vi "FGGA TCP Packet_v3.2.vi"(0 "ID":string, 5 "Version":string, 7 "TCP Packet In":string, 9 "utc_time":u32, 12 "Data Array":string[](array[string])) -> (8 "TCP Binary Packet":string)   [LabVIEW 2014]
panel:
  out "array":string[](array[string])
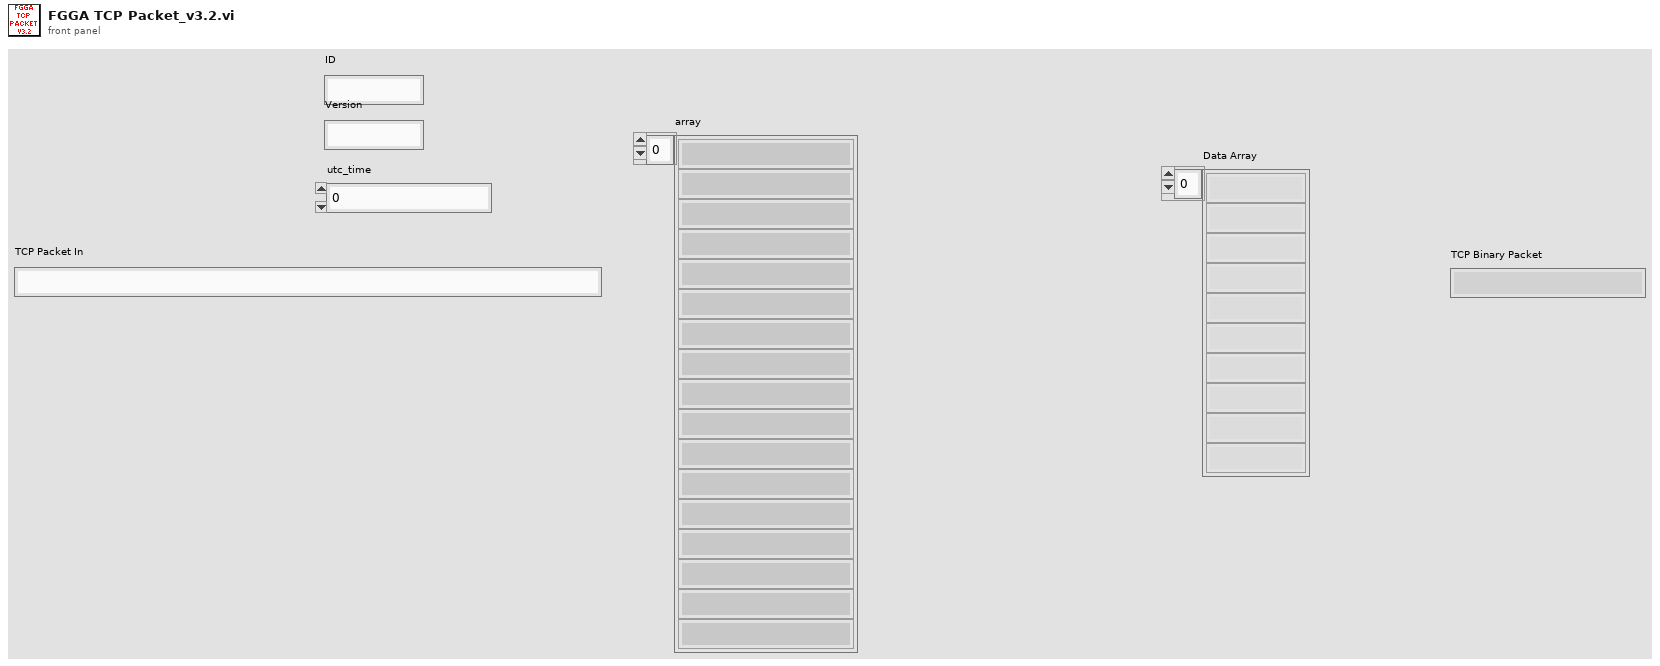
[diagram p1: front panel]
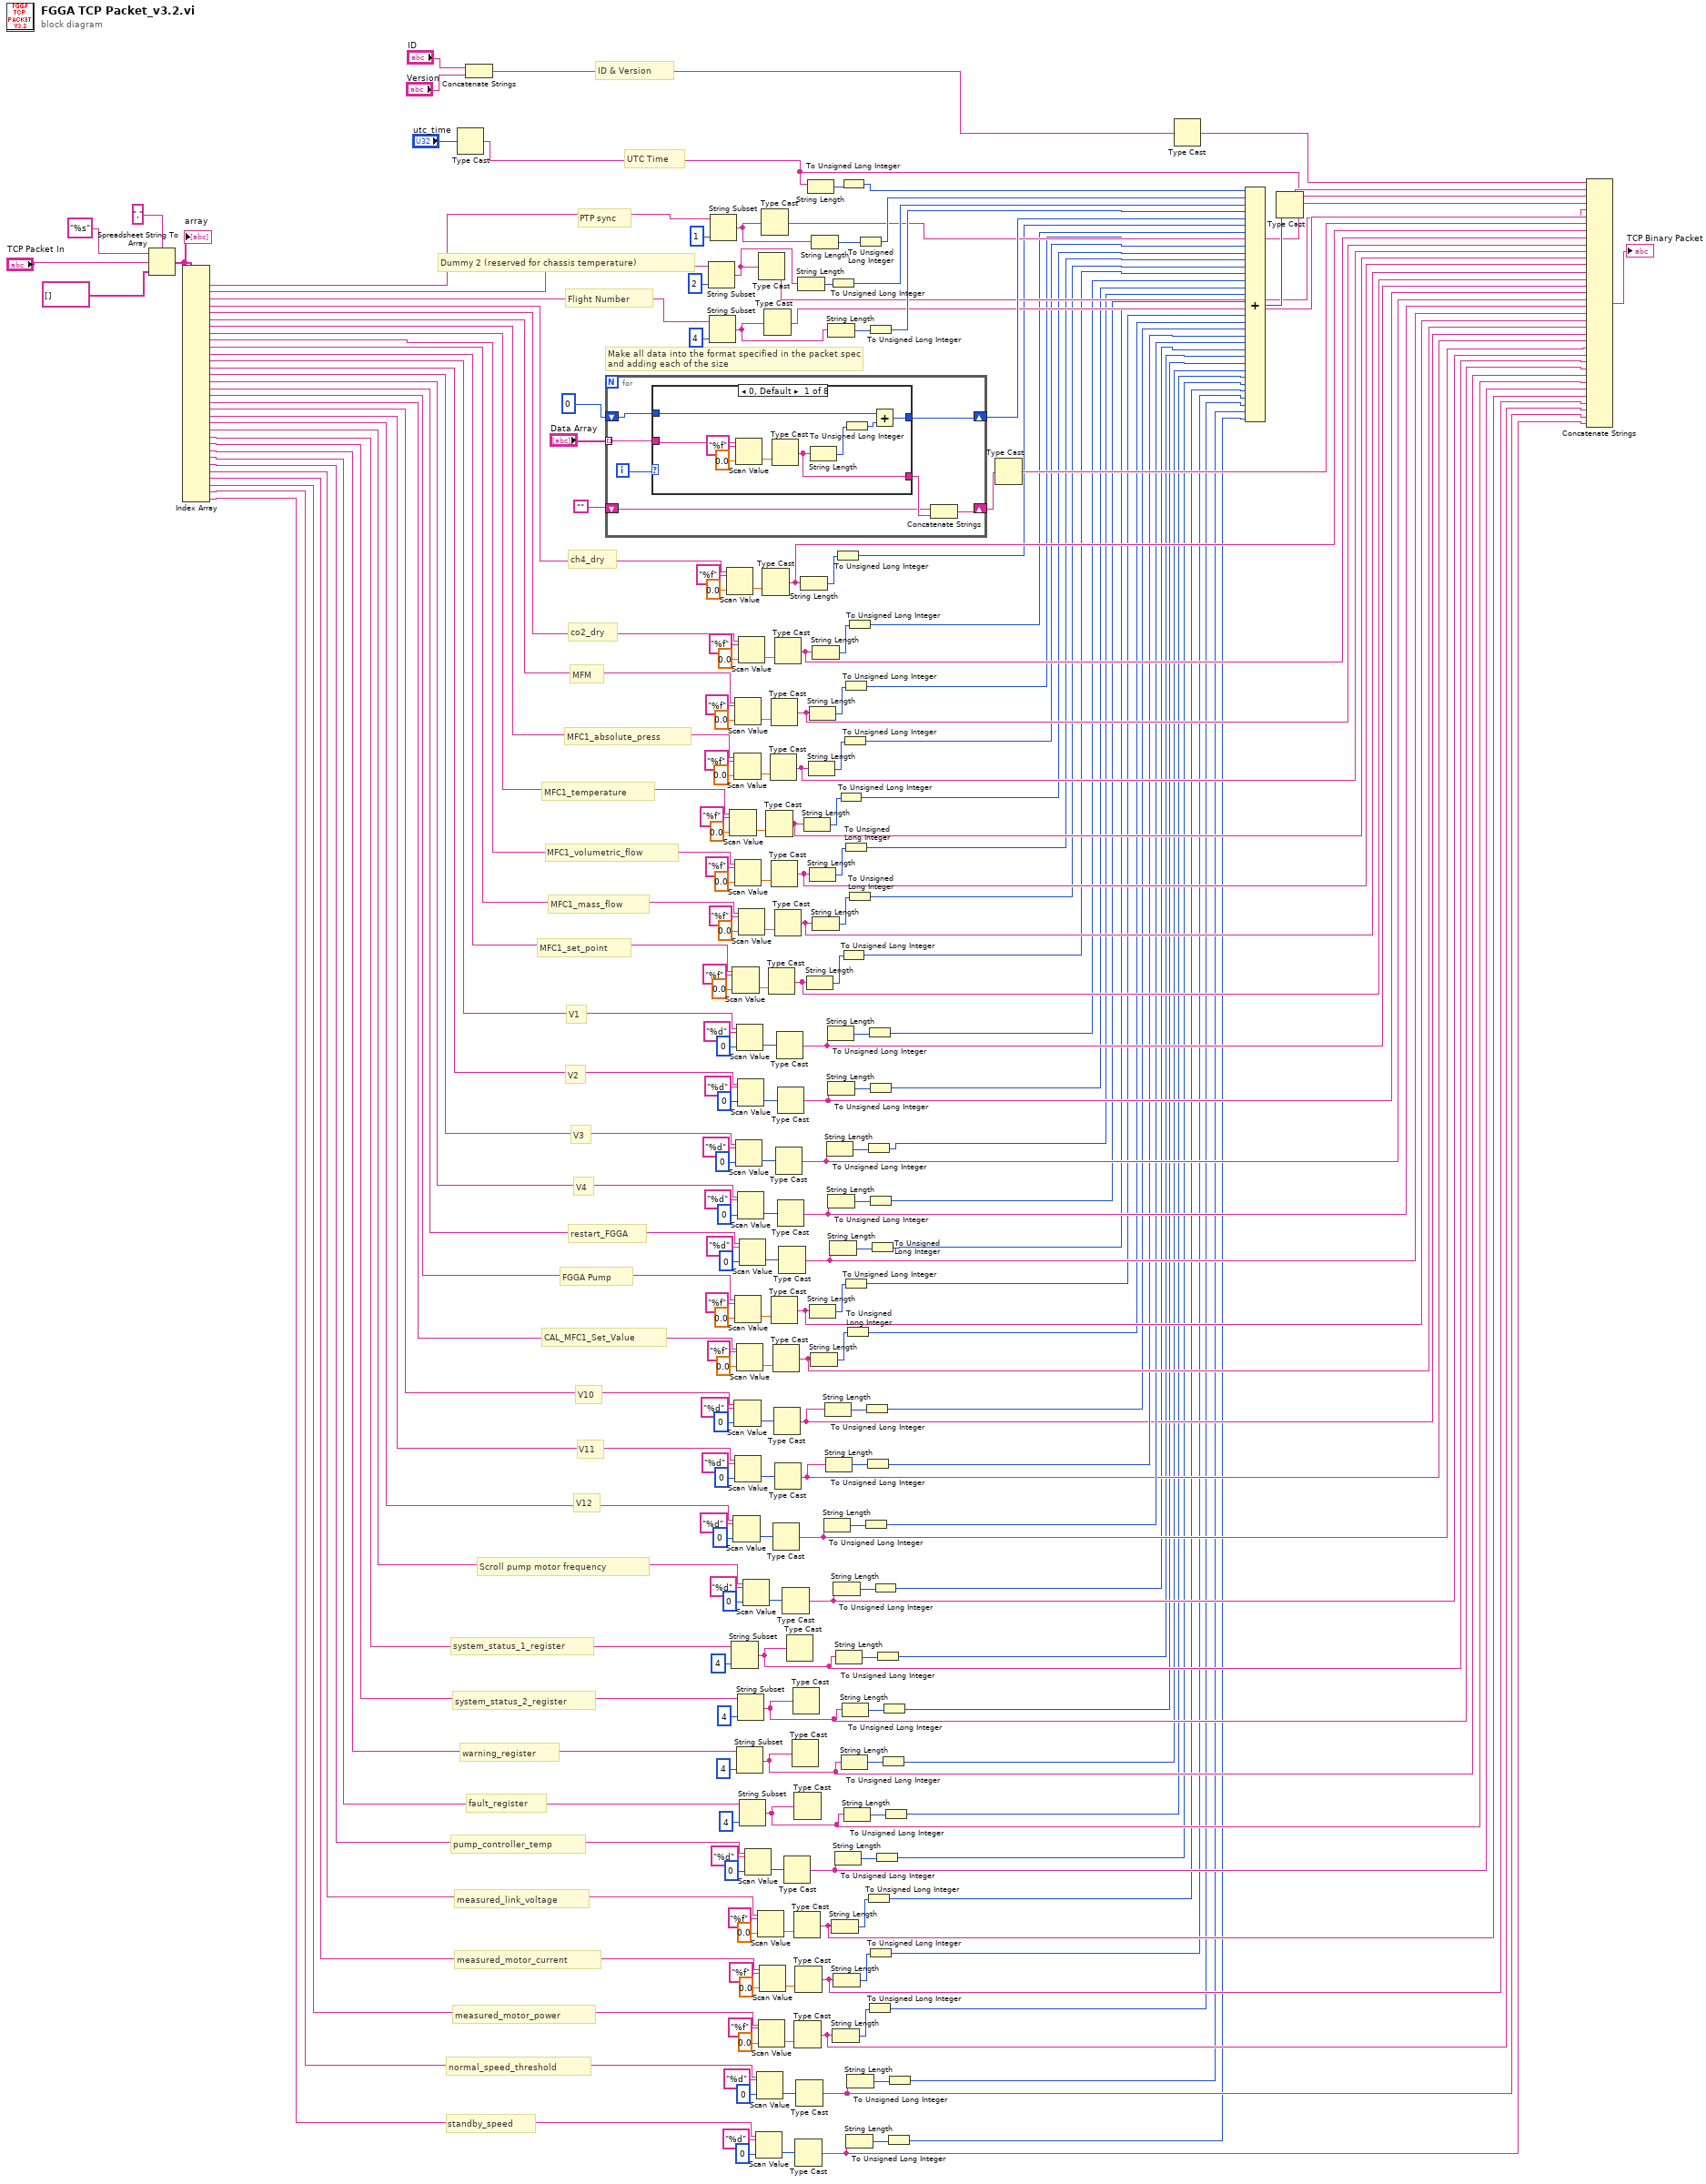
[diagram p0: block diagram]
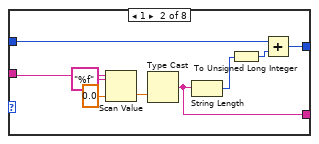
[diagram p2: hidden frame]
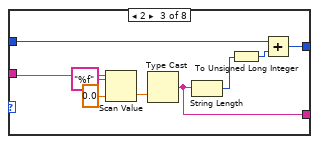
[diagram p3: hidden frame]
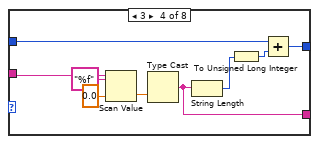
[diagram p4: hidden frame]
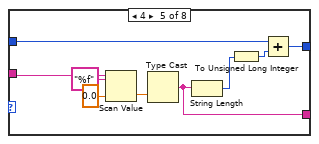
[diagram p5: hidden frame]
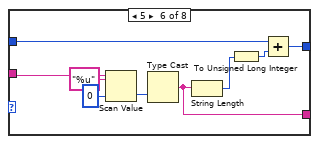
[diagram p6: hidden frame]
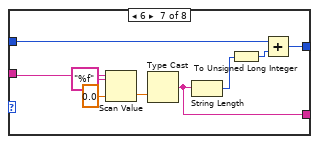
[diagram p7: hidden frame]
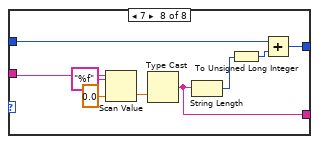
[diagram p8: hidden frame]
diagram:
  # "standby_speed"
  # "normal_speed_threshold"
  # "measured_motor_power"
  # "measured_motor_current"
  # "measured_link_voltage"
  # "pump_controller_temp"
  # "fault_register"
  # "warning_register"
  # "system_status_2_register"
  # "system_status_1_register"
  # "Scroll pump motor frequency"
  # "V12"
  # "V11"
  # "V10"
  # "PTP sync"
  # "CAL_MFC1_Set_Value"
  # "FGGA Pump"
  # "restart_FGGA"
  # "V4"
  # "V3"
  # "V2"
  # "V1"
  # "MFC1_set_point"
  # "MFC1_mass_flow"
  # "MFC1_volumetric_flow"
  # "MFC1_temperature"
  # "MFC1_absolute_press"
  # "MFM"
  # "co2_dry"
  # "ch4_dry"
  # "Flight Number"
  # "Dummy 2 (reserved for chassis temperature)"
  # "UTC Time"
  # "ID & Version"
  # "Make all data into the format specified in the packet spec\nand adding each of the size"
  n1 = Spreadsheet String To Array(delimiter (Tab)=",", format string="%s", spreadsheet string="TCP Packet In", array type (2D Dbl)=string[] []) -> (array=w192:string[])
  "array" <- w192
  n2 = Index Array(array=w192) -> (element #1=w191:string, element #2=w190:string, element #3=w189:string, element #4=w188:string, element #5=w187:string, element #6=w162:string, element #7=w159:string, element #8=w156:string, element #9=w153:string, element #10=w150:string, element #11=w147:string, element #12=w140:string, element #13=w133:string, element #14=w110:string, element #15=w107:string, element #16=w104:string, element #17=w101:string, element #18=w98:string, element #19=w78:string, element #20=w77:string, element #21=w76:string, element #22=w33:string, element #23=w32:string, element #24=w31:string, element #25=w30:string, element #26=w29:string, element #27=w28:string, element #28=w27:string, element #29=w26:string, element #30=w25:string, element #31=w24:string, element #32=w23:string)  [unwired: 32 in]
  n3 = Type Cast(x="utc_time") -> (*(type *) &x=w91:string)  [unwired: 1 in]
  n4 = Concatenate Strings("ID", "Version") -> (w93:string)
  n5 = for {
    tunnel: "Data Array" -> [w241] mode=indexing
    shift-right: [w239] -> w223
    shift-left: u32 0 -> [w240]
    shift-right: [w238] -> w212
    shift-left: "" -> [w236]
    i -> [w242]
    n6 = case shown="0, Default" w242 {
      tunnel: w241 -> [w249 w258 w267 w276 w285 w294 w303 w312]
      tunnel: w240 -> [w247 w256 w265 w274 w283 w292 w301 w310]
      tunnel: [w244 w253 w262 w271 w280 w289 w298 w307] -> w239
      tunnel: [w243 w252 w261 w270 w279 w288 w297 w306] -> w237
      frame 0, Default {
        n7 = Scan Value(string=w249, format string="%f", default (0 dbl)=sgl 0.0 ("default (0 I32)")) -> (value=w251:sgl)  [unwired: 1 out]
        n8 = Type Cast(x=w251) -> (*(type *) &x=w243:string)  [unwired: 1 in]
        n9 = String Length(string=w243) -> (length=w246:i32)
        n10 = To Unsigned Long Integer(number=w246) -> (unsigned 32bit integer=w245:u32)
        n11 = Add(x=w247, y=w245) -> (x+y=w244:u32)
      }
      frame 1 {
        n12 = Scan Value(string=w258, format string="%f", default (0 dbl)=sgl 0.0 ("default (0 I32)")) -> (value=w260:sgl)  [unwired: 1 out]
        n13 = Type Cast(x=w260) -> (*(type *) &x=w252:string)  [unwired: 1 in]
        n14 = String Length(string=w252) -> (length=w255:i32)
        n15 = To Unsigned Long Integer(number=w255) -> (unsigned 32bit integer=w254:u32)
        n16 = Add(x=w256, y=w254) -> (x+y=w253:u32)
      }
      frame 2 {
        n17 = Scan Value(string=w267, format string="%f", default (0 dbl)=sgl 0.0 ("default (0 I32)")) -> (value=w269:sgl)  [unwired: 1 out]
        n18 = Type Cast(x=w269) -> (*(type *) &x=w261:string)  [unwired: 1 in]
        n19 = String Length(string=w261) -> (length=w264:i32)
        n20 = To Unsigned Long Integer(number=w264) -> (unsigned 32bit integer=w263:u32)
        n21 = Add(x=w265, y=w263) -> (x+y=w262:u32)
      }
      frame 3 {
        n22 = Scan Value(string=w276, format string="%f", default (0 dbl)=sgl 0.0 ("default (0 I32)")) -> (value=w278:sgl)  [unwired: 1 out]
        n23 = Type Cast(x=w278) -> (*(type *) &x=w270:string)  [unwired: 1 in]
        n24 = String Length(string=w270) -> (length=w273:i32)
        n25 = To Unsigned Long Integer(number=w273) -> (unsigned 32bit integer=w272:u32)
        n26 = Add(x=w274, y=w272) -> (x+y=w271:u32)
      }
      frame 4 {
        n27 = Scan Value(string=w285, format string="%f", default (0 dbl)=sgl 0.0 ("default (0 I32)")) -> (value=w287:sgl)  [unwired: 1 out]
        n28 = Type Cast(x=w287) -> (*(type *) &x=w279:string)  [unwired: 1 in]
        n29 = String Length(string=w279) -> (length=w282:i32)
        n30 = To Unsigned Long Integer(number=w282) -> (unsigned 32bit integer=w281:u32)
        n31 = Add(x=w283, y=w281) -> (x+y=w280:u32)
      }
      frame 5 {
        n32 = Scan Value(string=w294, format string="%u", default (0 dbl)=u16 0 ("default (0 I32)")) -> (value=w296:u16)  [unwired: 1 out]
        n33 = Type Cast(x=w296) -> (*(type *) &x=w288:string)  [unwired: 1 in]
        n34 = String Length(string=w288) -> (length=w291:i32)
        n35 = To Unsigned Long Integer(number=w291) -> (unsigned 32bit integer=w290:u32)
        n36 = Add(x=w292, y=w290) -> (x+y=w289:u32)
      }
      frame 6 {
        n37 = Scan Value(string=w303, format string="%f", default (0 dbl)=sgl 0.0 ("default (0 I32)")) -> (value=w305:sgl)  [unwired: 1 out]
        n38 = Type Cast(x=w305) -> (*(type *) &x=w297:string)  [unwired: 1 in]
        n39 = String Length(string=w297) -> (length=w300:i32)
        n40 = To Unsigned Long Integer(number=w300) -> (unsigned 32bit integer=w299:u32)
        n41 = Add(x=w301, y=w299) -> (x+y=w298:u32)
      }
      frame 7 {
        n42 = Scan Value(string=w312, format string="%f", default (0 dbl)=sgl 0.0 ("default (0 I32)")) -> (value=w314:sgl)  [unwired: 1 out]
        n43 = Type Cast(x=w314) -> (*(type *) &x=w306:string)  [unwired: 1 in]
        n44 = String Length(string=w306) -> (length=w309:i32)
        n45 = To Unsigned Long Integer(number=w309) -> (unsigned 32bit integer=w308:u32)
        n46 = Add(x=w310, y=w308) -> (x+y=w307:u32)
      }
    }
    n47 = Concatenate Strings(w236, w237) -> (w238:string)
  }
  n48 = String Subset(string=w190, length (rest)=2 ("length (rest)")) -> (substring=w210:string)  [unwired: 1 in]
  n49 = String Subset(string=w189, length (rest)=4 ("length (rest)")) -> (substring=w216:string)  [unwired: 1 in]
  n50 = String Subset(string=w191, length (rest)=1 ("length (rest)")) -> (substring=w219:string)  [unwired: 1 in]
  n51 = Scan Value(string=w188, format string="%f", default (0 dbl)=sgl 0.0 ("default (0 I32)")) -> (value=w208:sgl)  [unwired: 1 out]
  n52 = Scan Value(string=w156, format string="%f", default (0 dbl)=sgl 0.0 ("default (0 I32)")) -> (value=w178:sgl)  [unwired: 1 out]
  n53 = String Subset(string=w32, length (rest)=4 ("length (rest)")) -> (substring=w19:string)  [unwired: 1 in]
  n54 = Scan Value(string=w147, format string="%f", default (0 dbl)=sgl 0.0 ("default (0 I32)")) -> (value=w166:sgl)  [unwired: 1 out]
  n55 = Scan Value(string=w76, format string="%d", default (0 dbl)=u16 0 ("default (0 I32)")) -> (value=w79:u16)  [unwired: 1 out]
  n56 = Scan Value(string=w159, format string="%f", default (0 dbl)=sgl 0.0 ("default (0 I32)")) -> (value=w182:sgl)  [unwired: 1 out]
  n57 = Scan Value(string=w78, format string="%d", default (0 dbl)=u16 0 ("default (0 I32)")) -> (value=w87:u16)  [unwired: 1 out]
  n58 = Scan Value(string=w162, format string="%f", default (0 dbl)=sgl 0.0 ("default (0 I32)")) -> (value=w186:sgl)  [unwired: 1 out]
  n59 = Scan Value(string=w153, format string="%f", default (0 dbl)=sgl 0.0 ("default (0 I32)")) -> (value=w174:sgl)  [unwired: 1 out]
  n60 = Scan Value(string=w101, format string="%f", default (0 dbl)=sgl 0.0 ("default (0 I32)")) -> (value=w118:sgl)  [unwired: 1 out]
  n61 = Scan Value(string=w77, format string="%d", default (0 dbl)=u16 0 ("default (0 I32)")) -> (value=w83:u16)  [unwired: 1 out]
  n62 = Scan Value(string=w110, format string="%d", default (0 dbl)=u16 0 ("default (0 I32)")) -> (value=w127:u16)  [unwired: 1 out]
  n63 = Scan Value(string=w140, format string="%d", default (0 dbl)=u16 0 ("default (0 I32)")) -> (value=w141:u16)  [unwired: 1 out]
  n64 = Scan Value(string=w98, format string="%f", default (0 dbl)=sgl 0.0 ("default (0 I32)")) -> (value=w114:sgl)  [unwired: 1 out]
  n65 = String Subset(string=w30, length (rest)=4 ("length (rest)")) -> (substring=w15:string)  [unwired: 1 in]
  n66 = Scan Value(string=w133, format string="%d", default (0 dbl)=u16 0 ("default (0 I32)")) -> (value=w134:u16)  [unwired: 1 out]
  n67 = Scan Value(string=w107, format string="%d", default (0 dbl)=u16 0 ("default (0 I32)")) -> (value=w123:u16)  [unwired: 1 out]
  n68 = String Subset(string=w31, length (rest)=4 ("length (rest)")) -> (substring=w17:string)  [unwired: 1 in]
  n69 = Scan Value(string=w187, format string="%f", default (0 dbl)=sgl 0.0 ("default (0 I32)")) -> (value=w202:sgl)  [unwired: 1 out]
  n70 = Scan Value(string=w150, format string="%f", default (0 dbl)=sgl 0.0 ("default (0 I32)")) -> (value=w170:sgl)  [unwired: 1 out]
  n71 = Scan Value(string=w104, format string="%d", default (0 dbl)=u16 0 ("default (0 I32)")) -> (value=w119:u16)  [unwired: 1 out]
  n72 = String Subset(string=w29, length (rest)=4 ("length (rest)")) -> (substring=w13:string)  [unwired: 1 in]
  n73 = Scan Value(string=w33, format string="%d", default (0 dbl)=u16 0 ("default (0 I32)")) -> (value=w66:u16)  [unwired: 1 out]
  n74 = Scan Value(string=w28, format string="%d", default (0 dbl)=u16 0 ("default (0 I32)")) -> (value=w54:u16)  [unwired: 1 out]
  n75 = Scan Value(string=w23, format string="%d", default (0 dbl)=u16 0 ("default (0 I32)")) -> (value=w34:u16)  [unwired: 1 out]
  n76 = Scan Value(string=w24, format string="%d", default (0 dbl)=u16 0 ("default (0 I32)")) -> (value=w38:u16)  [unwired: 1 out]
  n77 = Scan Value(string=w27, format string="%f", default (0 dbl)=sgl 0.0 ("default (0 I32)")) -> (value=w53:sgl)  [unwired: 1 out]
  n78 = Type Cast(x=w210) -> (*(type *) &x=w209:string)  [unwired: 1 in]
  n79 = Scan Value(string=w25, format string="%f", default (0 dbl)=sgl 0.0 ("default (0 I32)")) -> (value=w45:sgl)  [unwired: 1 out]
  n80 = Scan Value(string=w26, format string="%f", default (0 dbl)=sgl 0.0 ("default (0 I32)")) -> (value=w49:sgl)  [unwired: 1 out]
  n81 = Type Cast(x=w219) -> (*(type *) &x=w218:string)  [unwired: 1 in]
  n82 = Type Cast(x=w208) -> (*(type *) &x=w204:string)  [unwired: 1 in]
  n83 = Type Cast(x=w216) -> (*(type *) &x=w217:string)  [unwired: 1 in]
  n84 = Type Cast(x=w178) -> (*(type *) &x=w154:string)  [unwired: 1 in]
  n85 = Type Cast(x=w166) -> (*(type *) &x=w145:string)  [unwired: 1 in]
  n86 = Type Cast(x=w182) -> (*(type *) &x=w157:string)  [unwired: 1 in]
  n87 = Type Cast(x=w186) -> (*(type *) &x=w160:string)  [unwired: 1 in]
  n88 = Type Cast(x=w174) -> (*(type *) &x=w151:string)  [unwired: 1 in]
  n89 = Type Cast(x=w118) -> (*(type *) &x=w99:string)  [unwired: 1 in]
  n90 = Type Cast(x=w114) -> (*(type *) &x=w96:string)  [unwired: 1 in]
  n91 = Type Cast(x=w79) -> (*(type *) &x=w70:string)  [unwired: 1 in]
  n92 = Type Cast(x=w87) -> (*(type *) &x=w72:string)  [unwired: 1 in]
  n93 = Type Cast(x=w202) -> (*(type *) &x=w197:string)  [unwired: 1 in]
  n94 = Type Cast(x=w170) -> (*(type *) &x=w148:string)  [unwired: 1 in]
  n95 = Type Cast(x=w83) -> (*(type *) &x=w71:string)  [unwired: 1 in]
  n96 = Type Cast(x=w127) -> (*(type *) &x=w108:string)  [unwired: 1 in]
  n97 = Type Cast(x=w141) -> (*(type *) &x=w138:string)  [unwired: 1 in]
  n98 = Type Cast(x=w134) -> (*(type *) &x=w131:string)  [unwired: 1 in]
  n99 = Type Cast(x=w123) -> (*(type *) &x=w105:string)  [unwired: 1 in]
  n100 = Type Cast(x=w119) -> (*(type *) &x=w102:string)  [unwired: 1 in]
  n101 = Type Cast(x=w66) -> (*(type *) &x=w21:string)  [unwired: 1 in]
  n102 = Type Cast(x=w54) -> (*(type *) &x=w11:string)  [unwired: 1 in]
  n103 = Type Cast(x=w19) -> ()  [unwired: 1 in, 1 out]
  n104 = Type Cast(x=w15) -> ()  [unwired: 1 in, 1 out]
  n105 = Type Cast(x=w17) -> ()  [unwired: 1 in, 1 out]
  n106 = Type Cast(x=w53) -> (*(type *) &x=w9:string)  [unwired: 1 in]
  n107 = Type Cast(x=w13) -> ()  [unwired: 1 in, 1 out]
  n108 = Type Cast(x=w45) -> (*(type *) &x=w5:string)  [unwired: 1 in]
  n109 = Type Cast(x=w49) -> (*(type *) &x=w7:string)  [unwired: 1 in]
  n110 = Type Cast(x=w34) -> (*(type *) &x=w1:string)  [unwired: 1 in]
  n111 = Type Cast(x=w38) -> (*(type *) &x=w3:string)  [unwired: 1 in]
  n112 = String Length(string=w210) -> (length=w230:i32)
  n113 = String Length(string=w204) -> (length=w205:i32)
  n114 = String Length(string=w154) -> (length=w175:i32)
  n115 = String Length(string=w145) -> (length=w163:i32)
  n116 = String Length(string=w91) -> (length=w235:i32)
  n117 = String Length(string=w157) -> (length=w179:i32)
  n118 = String Length(string=w160) -> (length=w183:i32)
  n119 = String Length(string=w151) -> (length=w171:i32)
  n120 = String Length(string=w99) -> (length=w115:i32)
  n121 = String Length(string=w96) -> (length=w111:i32)
  n122 = String Length(string=w219) -> (length=w232:i32)
  n123 = String Length(string=w197) -> (length=w199:i32)
  n124 = String Length(string=w148) -> (length=w167:i32)
  n125 = String Length(string=w70) -> (length=w82:i32)
  n126 = String Length(string=w72) -> (length=w90:i32)
  n127 = String Length(string=w71) -> (length=w86:i32)
  n128 = String Length(string=w108) -> (length=w130:i32)
  n129 = String Length(string=w138) -> (length=w144:i32)
  n130 = String Length(string=w216) -> (length=w227:i32)
  n131 = String Length(string=w131) -> (length=w137:i32)
  n132 = String Length(string=w105) -> (length=w126:i32)
  n133 = To Unsigned Long Integer(number=w230) -> (unsigned 32bit integer=w229:u32)
  n134 = String Length(string=w102) -> (length=w122:i32)
  n135 = String Length(string=w9) -> (length=w50:i32)
  n136 = String Length(string=w5) -> (length=w42:i32)
  n137 = String Length(string=w21) -> (length=w69:i32)
  n138 = String Length(string=w7) -> (length=w46:i32)
  n139 = To Unsigned Long Integer(number=w205) -> (unsigned 32bit integer=w203:u32)
  n140 = String Length(string=w11) -> (length=w57:i32)
  n141 = String Length(string=w19) -> (length=w64:i32)
  n142 = To Unsigned Long Integer(number=w175) -> (unsigned 32bit integer=w155:u32)
  n143 = To Unsigned Long Integer(number=w235) -> (unsigned 32bit integer=w234:u32)
  n144 = To Unsigned Long Integer(number=w163) -> (unsigned 32bit integer=w146:u32)
  n145 = String Length(string=w15) -> (length=w60:i32)
  n146 = To Unsigned Long Integer(number=w179) -> (unsigned 32bit integer=w158:u32)
  n147 = String Length(string=w17) -> (length=w62:i32)
  n148 = To Unsigned Long Integer(number=w183) -> (unsigned 32bit integer=w161:u32)
  n149 = To Unsigned Long Integer(number=w171) -> (unsigned 32bit integer=w152:u32)
  n150 = To Unsigned Long Integer(number=w115) -> (unsigned 32bit integer=w100:u32)
  n151 = String Length(string=w13) -> (length=w58:i32)
  n152 = To Unsigned Long Integer(number=w111) -> (unsigned 32bit integer=w97:u32)
  n153 = To Unsigned Long Integer(number=w199) -> (unsigned 32bit integer=w198:u32)
  n154 = To Unsigned Long Integer(number=w167) -> (unsigned 32bit integer=w149:u32)
  n155 = String Length(string=w1) -> (length=w37:i32)
  n156 = String Length(string=w3) -> (length=w41:i32)
  n157 = To Unsigned Long Integer(number=w232) -> (unsigned 32bit integer=w231:u32)
  n158 = To Unsigned Long Integer(number=w82) -> (unsigned 32bit integer=w73:u32)
  n159 = To Unsigned Long Integer(number=w90) -> (unsigned 32bit integer=w75:u32)
  n160 = To Unsigned Long Integer(number=w86) -> (unsigned 32bit integer=w74:u32)
  n161 = To Unsigned Long Integer(number=w130) -> (unsigned 32bit integer=w109:u32)
  n162 = To Unsigned Long Integer(number=w50) -> (unsigned 32bit integer=w10:u32)
  n163 = To Unsigned Long Integer(number=w144) -> (unsigned 32bit integer=w139:u32)
  n164 = To Unsigned Long Integer(number=w42) -> (unsigned 32bit integer=w6:u32)
  n165 = To Unsigned Long Integer(number=w227) -> (unsigned 32bit integer=w226:u32)
  n166 = To Unsigned Long Integer(number=w137) -> (unsigned 32bit integer=w132:u32)
  n167 = To Unsigned Long Integer(number=w126) -> (unsigned 32bit integer=w106:u32)
  n168 = To Unsigned Long Integer(number=w46) -> (unsigned 32bit integer=w8:u32)
  n169 = To Unsigned Long Integer(number=w122) -> (unsigned 32bit integer=w103:u32)
  n170 = To Unsigned Long Integer(number=w69) -> (unsigned 32bit integer=w22:u32)
  n171 = To Unsigned Long Integer(number=w57) -> (unsigned 32bit integer=w12:u32)
  n172 = To Unsigned Long Integer(number=w64) -> (unsigned 32bit integer=w20:u32)
  n173 = To Unsigned Long Integer(number=w60) -> (unsigned 32bit integer=w16:u32)
  n174 = To Unsigned Long Integer(number=w62) -> (unsigned 32bit integer=w18:u32)
  n175 = To Unsigned Long Integer(number=w58) -> (unsigned 32bit integer=w14:u32)
  n176 = To Unsigned Long Integer(number=w37) -> (unsigned 32bit integer=w2:u32)
  n177 = To Unsigned Long Integer(number=w41) -> (unsigned 32bit integer=w4:u32)
  n178 = Type Cast(x=w212) -> (*(type *) &x=w215:string)  [unwired: 1 in]
  n179 = Type Cast(x=w93) -> (*(type *) &x=w222:string)  [unwired: 1 in]
  n180 = Compound Arithmetic op=ADD(w234, w231, w229, w226, w223, w203, w198, w161, w158, w155, w152, w149, w146, w139, w132, w109, w106, w103, w100, w97, w75, w74, w73, w22, w20, w18, w16, w14, w12, w10, w8, w6, w4, w2) -> (w221:u32)
  n181 = Type Cast(x=w221) -> (*(type *) &x=w220:string)  [unwired: 1 in]
  n182 = Concatenate Strings(w222, w220, w91, w218, w209, w217, w215, w204, w197, w160, w157, w154, w151, w148, w145, w138, w131, w108, w105, w102, w99, w96, w72, w71, w70, w21, w19, w17, w15, w13, w11, w9, w7, w5, w3, w1) -> (→"TCP Binary Packet":string)
